vi "Clear Table.vi"(8 "error in (no error)":errorcluster, 11 "Result Table.lvclass":refnum<class "Result Table.lvclass">) -> (0 "error out":errorcluster, 3 "Result Table":refnum<class "Result Table.lvclass">)   [LabVIEW 2020]
uses:
  Result Table.lvclass
  Result Table.lvclass/Result Table.ctl
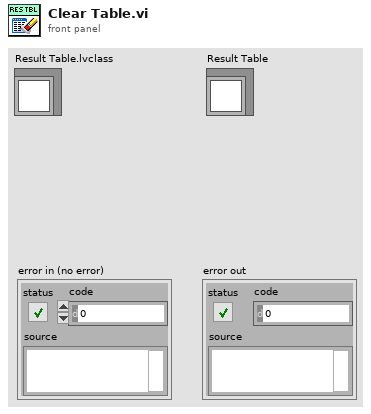
[diagram p1: front panel]
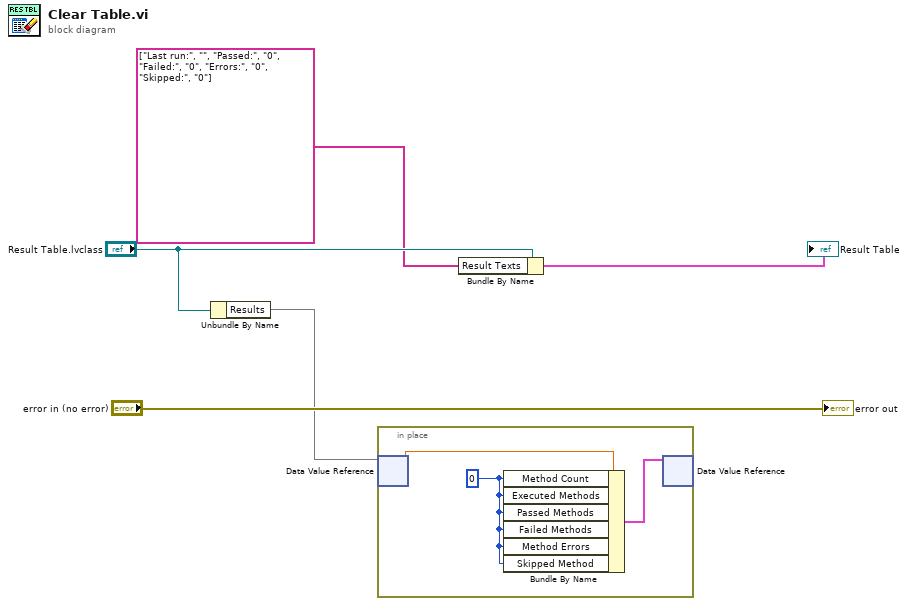
[diagram p0: block diagram]
diagram:
  n1 = Unbundle By Name("Result Table.lvclass") -> ("Results"=w3)
  n2 = in-place {
    w7 = u32 0 ("Method Count")
    n3 = in-place-dvr #1(w3) -> (w8:dbl)  [unwired: 1 out]
    n4 = Bundle By Name(cluster=w8, "Method Count"=w7, "Executed Methods"=w7, "Passed Methods"=w7, "Failed Methods"=w7, "Method Errors"=w7, "Skipped Method"=w7) -> (w6:cluster{})
    n5 = in-place-dvr #1(w6) -> ()  [unwired: 2 out]
  }
  n6 = Bundle By Name(cluster="Result Table.lvclass", "Result Texts"=string[] ["Last run:", "", "Passed:", "0", "Failed:", "0", "Errors:", "0", "Skipped:", "0"]) -> (→"Result Table":cluster{})
  "error out" <- "error in (no error)"
